vi "Open Wrapper.vi"(8 "error in (no error)":errorcluster) -> (0 "error out":errorcluster, 3 "Session":i64)   [LabVIEW 2021, in "Zenoh.lvclass"]
uses:
  Zenoh.lvclass
  typedef/Zenoh Errors.ctl
  <vilib>/CIF Foundation/CIF Utilities/Errors/Append Error Location.vi
  Zenoh.lvclass/Zenoh.ctl
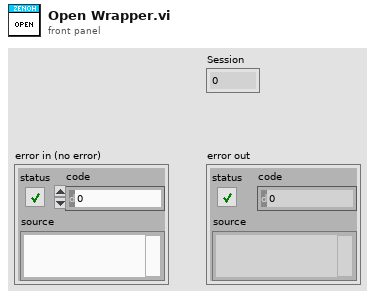
[diagram p1: front panel]
types:
  T1 = typedef "Zenoh.lvclass/Zenoh Errors.ctl" = enum16{"Open Session Error", "Open Subscription Error"}
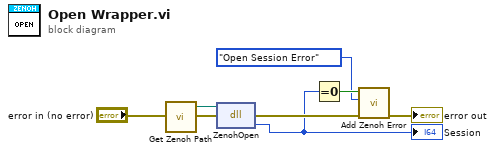
[diagram p0: block diagram]
diagram:
  n1 = call "Get Zenoh Path.vi"() -> ("Library Path"=w7:path)  [unwired: 4 in]
  n2 = dll-call lib="D:/dev/zenoh/wrapper/zenoh_wrapper_reader.dll" fn="ZenohOpen"(path in=w7, error in="error in (no error)") -> (error out=w5:errorcluster, "return type"=w2:i64)  [unwired: 1 in, 1 out]
  "Session" <- w2
  n3 = Equal To 0?(x=w2) -> (x = 0?=w3:bool)
  n4 = call "Add Zenoh Error.vi"("error in (no error)"=w5, "Error"=Zenoh_Errors."Open Session Error", "Insert Error"=w3) -> ("error out"=→"error out":errorcluster)  [unwired: 8 in]
